vi "2DStyle.vi"(10 "Style":T1) -> (2 "Style":u8)   [LabVIEW 2020]
uses:
  _Controls/Style.ctl
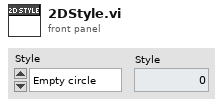
[diagram p1: front panel]
types:
  T1 = typedef "Style.ctl" = enum16{"Empty circle", "Full circle", "Empty square", "Full square", "Cross"}
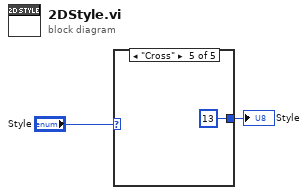
[diagram p0: block diagram]
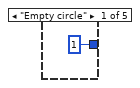
[diagram p2: hidden frame]
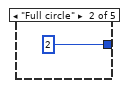
[diagram p3: hidden frame]
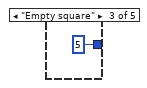
[diagram p4: hidden frame]
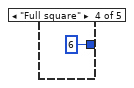
[diagram p5: hidden frame]
diagram:
  n1 = case shown="\"Cross\"" "Style" {
    tunnel: [u8 1 u8 2 u8 5 u8 6 u8 13] -> w1
    frame "Empty circle" {
    }
    frame "Full circle" {
    }
    frame "Empty square" {
    }
    frame "Full square" {
    }
    frame "Cross" {
    }
  }
  "Style" <- w1
